vi "SbigRegisterCCD.vi"(1 "GetDriverHandle":u16[](array[numeric]), 2 "GetCCDInfo":u16[](array[numeric])) -> (0 "CCD":T1)   [LabVIEW 2009]
uses:
  Controls/SbigReference.ctl
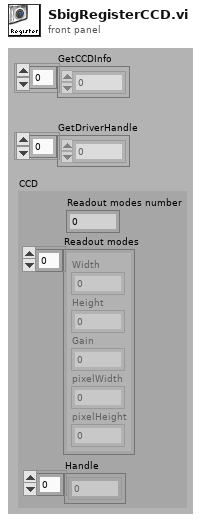
[diagram p1: front panel]
types:
  T1 = typedef "SbigReference.ctl" = cluster{"Readout modes number":u16, "Readout modes":cluster{"Width":u16, "Height":u16, "Gain":dbl, "pixelWidth":dbl, "pixelHeight":dbl}[], "Handle":u16[]}
  T2 = cluster{"Width":u16, "Height":u16, "Gain":dbl, "pixelWidth":dbl, "pixelHeight":dbl}
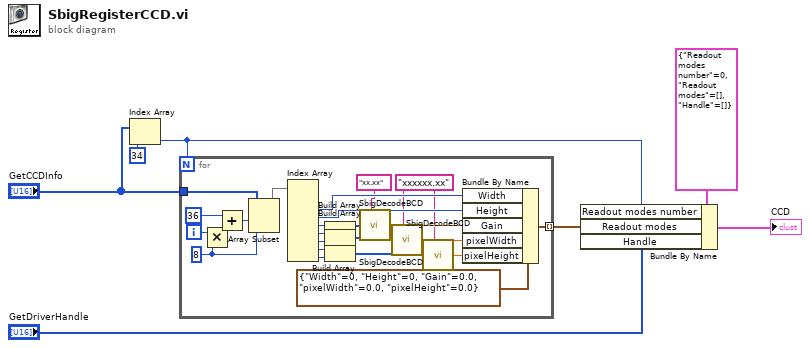
[diagram p0: block diagram]
diagram:
  n1 = Index Array(array="GetCCDInfo", index=34 ("Indice")) -> (element=w5:u16)
  n2 = for {
    N: w5 -> [_]
    tunnel: "GetCCDInfo" -> [w28]
    tunnel: [w21] -> w3 mode=indexing
    i -> [w31]
    w8 = "xxxxxx.xx" ("Format")
    w26 = 8 ("y")
    n3 = Multiply(x=w31, y=w26) -> (x*y=w30:i32)
    n4 = Add(x=36, y=w30) -> (x+y=w27:i32)
    n5 = Array Subset(array=w28, index=w27, length=w26) -> (w25:u16[])
    n6 = Index Array(array=w25) -> (element #2=w22:u16, element #3=w23:u16, element #4=w19:u16, element #5=w16:u16, element #6=w15:u16, element #7=w14:u16, element #8=w13:u16)  [unwired: 8 in, 1 out]
    n7 = Build Array(w19) -> (w20:u16[])
    n8 = Build Array(w16, w15) -> (w10:u16[])
    n9 = Build Array(w14, w13) -> (w9:u16[])
    n10 = call "SbigDecodeBCD.vi"("Format"="xx.xx", "Array of U16"=w20) -> ("nombre"=w18:dbl)  [unwired: 7 out]
    n11 = call "SbigDecodeBCD.vi"("Format"=w8, "Array of U16"=w10) -> ("nombre"=w12:dbl)  [unwired: 7 out]
    n12 = call "SbigDecodeBCD.vi"("Format"=w8, "Array of U16"=w9) -> ("nombre"=w11:dbl)  [unwired: 7 out]
    n13 = Bundle By Name(cluster=T2 {"Width"=0, "Height"=0, "Gain"=0.0, "pixelWidth"=0.0, "pixelHeight"=0.0}, "Width"=w22, "Height"=w23, "Gain"=w18, "pixelWidth"=w12, "pixelHeight"=w11) -> (w21:T2)
  }
  n14 = Bundle By Name(cluster=T1 {"Readout modes number"=0, "Readout modes"=[], "Handle"=[]} ("SbigReference"), "Readout modes number"=w5, "Readout modes"=w3, "Handle"="GetDriverHandle") -> (→"CCD":T1)
